vi "Parse In String (offset).vi"(10 "offset":i32, 11 "JSON (quote at offset)":string) -> (2 "offset":i32, 3 "String (incl quotes)":string)   [LabVIEW 2020, in "Library Commun.lvlib" / "JSON Value.lvclass"]
doc: "Parse out a JSON String (properly escaped) from the front of the incoming JSON fragment (must have a quote as first char)."
uses:
  JSON Value/JSON Value.lvclass
  JSON Value/JSON Value.lvclass/JSON Value.ctl
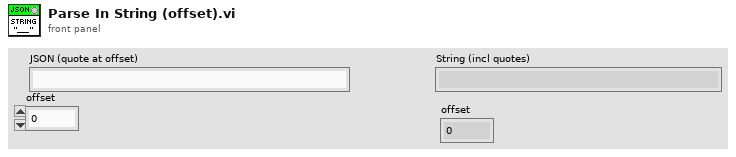
[diagram p1: front panel]
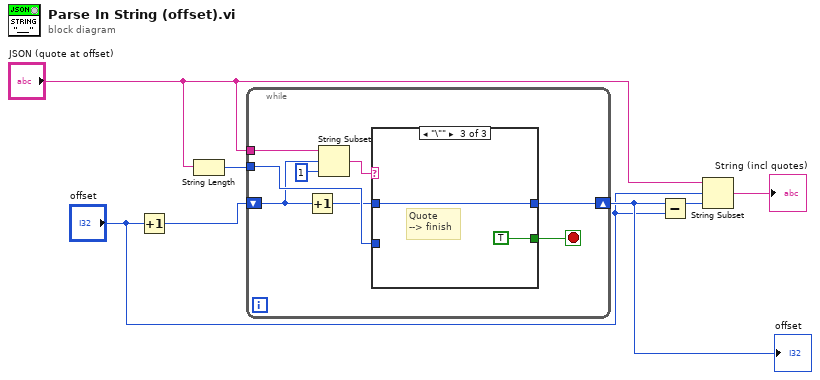
[diagram p0: block diagram]
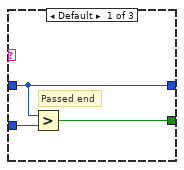
[diagram p2: hidden frame]
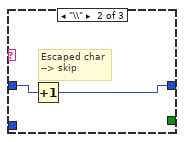
[diagram p3: hidden frame]
diagram:
  n1 = Increment(x="offset") -> (x+1=w3:i32)
  n2 = String Length(string="JSON (quote at offset)") -> (length=w5:i32)
  n3 = while {
    tunnel: "JSON (quote at offset)" -> [w15]
    shift-right: [w12] -> w6
    shift-left: w3 -> [w8]
    tunnel: w5 -> [w11]
    stop <- w10 stop-if-true
    n4 = Increment(x=w8) -> (x+1=w9:i32)
    n5 = String Subset(string=w15, offset (0)=w8, length (rest)=1 ("length (rest)")) -> (substring=w13:string)
    n6 = case shown="\"\\\"\"" w13 {
      tunnel: w9 -> [w18 w20 w22]
      tunnel: [w18 w19 w22] -> w12
      tunnel: w11 -> [w17 _ _]
      tunnel: [w16 _ TRUE] -> w10
      frame Default {
        # "Passed end"
        n7 = Greater?(x=w18, y=w17) -> (0:w16:bool)
      }
      frame "\\" {
        # "Escaped char\n--> skip"
        n8 = Increment(x=w20) -> (x+1=w19:i32)
      }
      frame "\"" {
        # "Quote\n--> finish"
      }
    }
  }
  "offset" <- w6
  n9 = Subtract(x=w6, y="offset") -> (x-y=w2:i32)
  n10 = String Subset(string="JSON (quote at offset)", offset (0)="offset", length (rest)=w2) -> (substring=→"String (incl quotes)":string)
